vi "Image path to image refnum.vi"(7 "Image to Add [ ]":T2 {"Scale" format="%#_g %"}, 11 "error in (no error)":errorcluster) -> (8 "Image to Add refnum [ ]":T1, 15 "error out":errorcluster)   [LabVIEW 2019, in "Exaprom PDF.lvlib"]
doc: "Version 1.0\nDeveloped by Jean-Marc Simard\nCopyright © 2010, Exaprom Inc.\nAll rights reserved.\nLicense: BSD\n\nWith iTextSharp 4.1.6 (http://itextsharp.sourceforge.net)\nunder Mozilla Public License Version 1.1\n(http://www.mozilla.org/MPL/MPL-1.1.html)"
uses:
  Controls/General Controls/Image to Add [ ].ctl
  Controls/Image Controls/Image Scale.ctl
  Controls/General Controls/Image to Add refnum [ ].ctl
  C:/work/niobrara_lv/labview pdf writer fixing/DLL/itextsharp.dll
  DLL/itextsharp.dll
  Exaprom PDF.lvlib
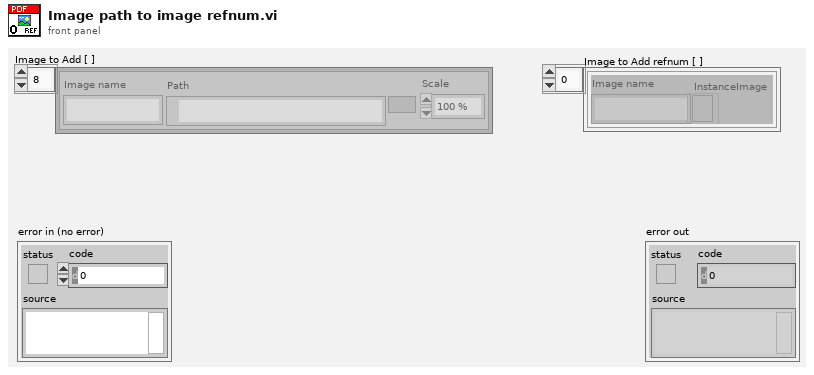
[diagram p1: front panel]
types:
  T1 = typedef "Exaprom PDF.lvlib/Image to Add refnum [ ].ctl" = cluster{"Image name":string, "InstanceImage":refnum<k24>}[]
  T2 = typedef "Exaprom PDF.lvlib/Image to Add [ ].ctl" = cluster{"Image name":string, "Path":path, "Scale":T3}[]
  T3 = typedef "Exaprom PDF.lvlib/Image Scale.ctl" = sgl
  T4 = cluster{"Image name":string, "InstanceImage":refnum<k24>}[]
  T5 = cluster{"Image name":string, "GetInstance":refnum<k24>}
  T6 = cluster{"Image name":string, "GetInstance":refnum<k24>}[]
  T7 = cluster{"Image name":string, "image":refnum<k24>}[]
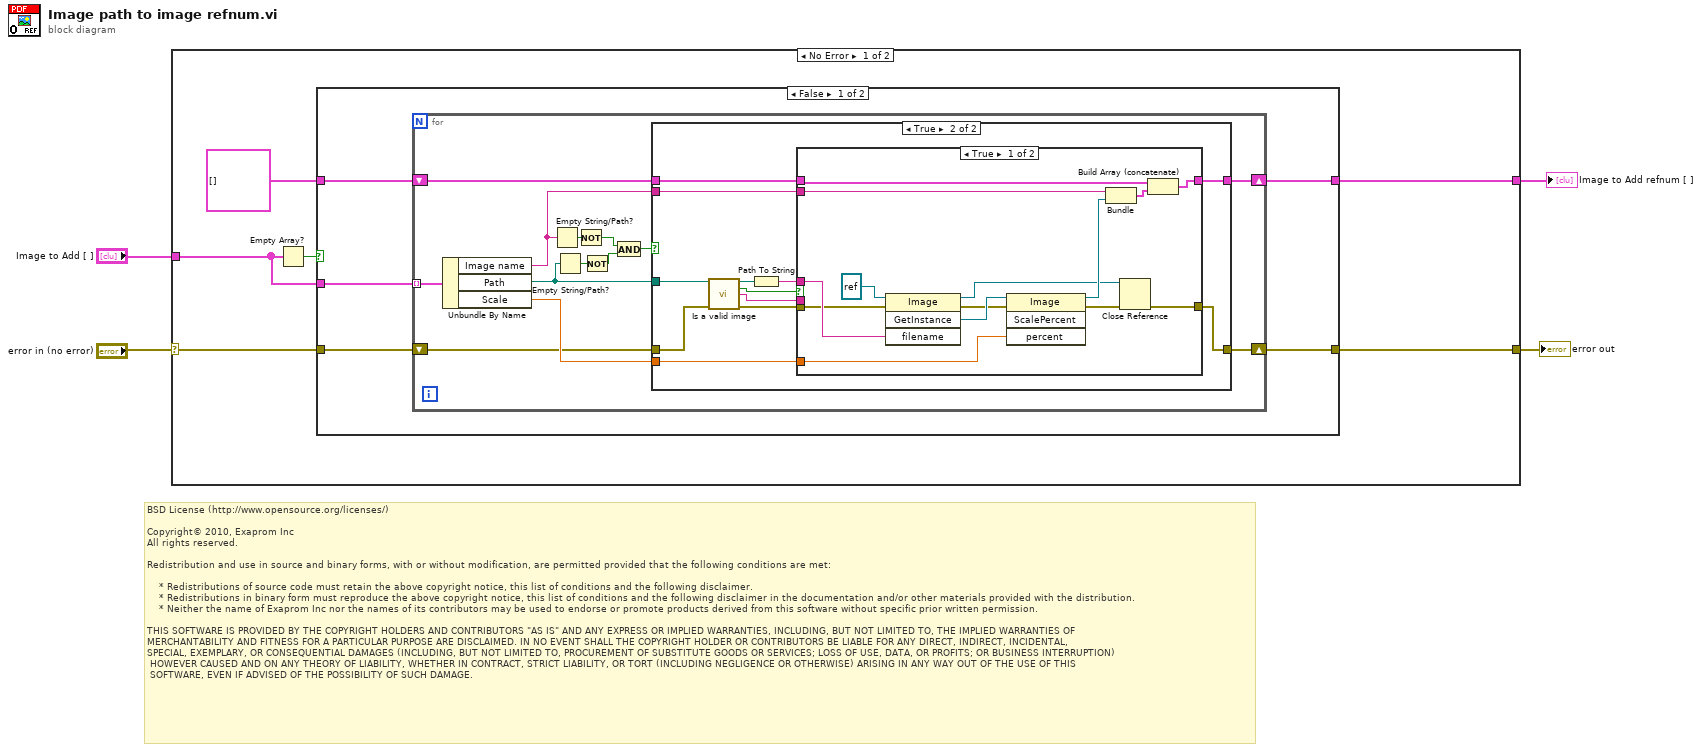
[diagram p0: block diagram]
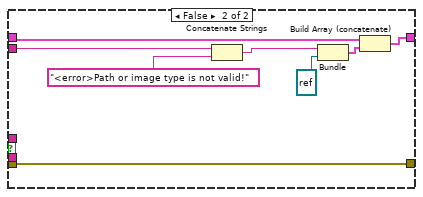
[diagram p3: hidden frame]
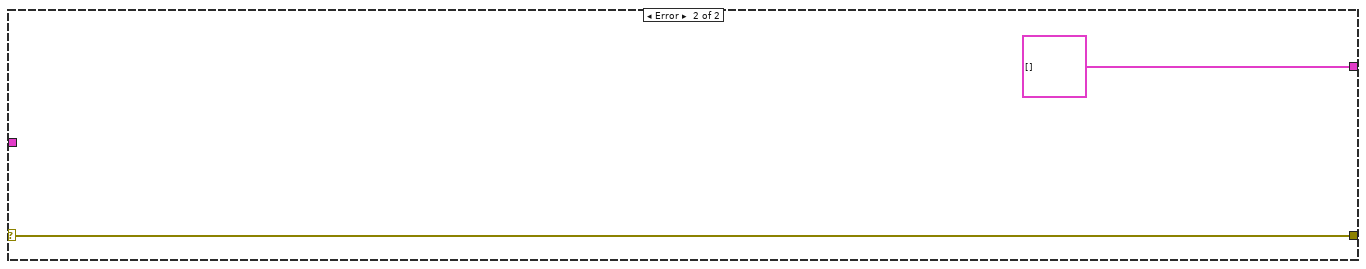
[diagram p5: hidden frame]
diagram:
  # "BSD License (http://www.opensource.org/licenses/)\n\nCopyright© 2010, Exaprom Inc\nAll rights reserved.\n\nRedistribution and use in source and binary forms, with or without modification, are permitted provided that the following conditions are met:\n\n    * Redistributions of source code must retain the above copyright notice, this list of conditions and the following disclaimer.\n    * Redistributions in binary form must reproduce the above copyright notice, this list of conditions and the following disclaimer in the documentation and/or other materials provided with the distribution.\n    * Neither the name of Exaprom Inc nor the names of its contributors may be used to endorse or promote products derived from this software without specific prior written permission.\n\nTHIS SOFTWARE IS PROVIDED BY THE COPYRIGHT HOLDERS AND CONTRIBUTORS \"AS IS\" AND ANY EXPRESS OR IMPLIED WARRANTIES, INCLUDING, BUT NOT LIMITED TO, THE IMPLIED WARRANTIES OF \nMERCHANTABILITY AND FITNESS FOR A PARTICULAR PURPOSE ARE DISCLAIMED. IN NO EVENT SHALL THE COPYRIGHT HOLDER OR CONTRIBUTORS BE LIABLE FOR ANY DIRECT, INDIRECT, INCIDENTAL,\nSPECIAL, EXEMPLARY, OR CONSEQUENTIAL DAMAGES (INCLUDING, BUT NOT LIMITED TO, PROCUREMENT OF SUBSTITUTE GOODS OR SERVICES; LOSS OF USE, DATA, OR PROFITS; OR BUSINESS INTERRUPTION)\n HOWEVER CAUSED AND ON ANY THEORY OF LIABILITY, WHETHER IN CONTRACT, STRICT LIABILITY, OR TORT (INCLUDING NEGLIGENCE OR OTHERWISE) ARISING IN ANY WAY OUT OF THE USE OF THIS\n SOFTWARE, EVEN IF ADVISED OF THE POSSIBILITY OF SUCH DAMAGE."
  n1 = case shown="No Error" "error in (no error)" {
    selector: "error in (no error)" -> [w5 w68]
    tunnel: "Image to Add [ ]" -> [w8 _]
    tunnel: [w7 w68] -> w2
    tunnel: [w6 T4 [] ("Image to Add [ ]")] -> w1
    frame No Error {
      n2 = Empty Array?(array=w8) -> (empty?=w9:bool)
      n3 = case shown="False" w9 {
        tunnel: w8 -> [w15 _]
        tunnel: T4 [] ("Image to Add [ ]") -> [w14 w66]
        tunnel: [w13 w66] -> w6
        tunnel: [w12 w65] -> w7
        tunnel: w5 -> [w11 w65]
        frame False {
          n4 = for {
            tunnel: w15 -> [w28] mode=indexing
            shift-right: [w21] -> w13
            shift-left: w14 -> [w22]
            shift-right: [w19] -> w12
            shift-left: w11 -> [w20]
            n5 = Unbundle By Name(w28) -> ("Image name"=w18:string, "Path"=w27:path, "Scale"=w23:T3)
            n6 = Empty String/Path?(string/path=w18) -> (empty?=w25:bool)
            n7 = Empty String/Path?(string/path=w27) -> (empty?=w26:bool)
            n8 = Not(x=w25) -> (.not. x?=w17:bool)
            n9 = Not(x=w26) -> (.not. x?=w16:bool)
            n10 = And(x=w17, y=w16) -> (x .and. y?=w24:bool)
            n11 = case shown="True" w24 {
              tunnel: w27 -> [_ w41]
              tunnel: w23 -> [_ w39]
              tunnel: w22 -> [w30 w37]
              tunnel: [w30 w36] -> w21
              tunnel: w20 -> [w29 w31]
              tunnel: [w29 w38] -> w19
              tunnel: w18 -> [_ w35]
              frame False {
              }
              frame True {
                n12 = call "Is a valid image.vi"("Image path"=w41, "error in (no error)"=w31) -> ("dup path"=w42:path, "Valid Image?"=w33:bool, "Message"=w32:string, "error out"=w34:errorcluster)  [unwired: 10 out]
                n13 = Path To String(path=w42) -> (string=w40:string)
                n14 = case shown="True" w33 {
                  tunnel: w40 -> [w54 _]
                  tunnel: w39 -> [w53 _]
                  tunnel: [w46 w60] -> w38
                  tunnel: w37 -> [w52 w64]
                  tunnel: [w51 w63] -> w36
                  tunnel: w35 -> [w49 w62]
                  tunnel: w34 -> [w43 w60]
                  tunnel: w32 -> [_ _]
                  frame True {
                    n15 = invoke class="Image" method="GetInstance"(reference=refnum<k24> refnum ("image"), error in=w43, "filename"=w54) -> (reference out=w45:refnum<k24>, error out=w55:errorcluster, "GetInstance"=w56:refnum<k24>)  [unwired: 1 in, 1 out]
                    n16 = invoke class="Image" method="ScalePercent"(reference=w56, error in=w55, "percent"=w53) -> (reference out=w50:refnum<k24>, error out=w47:errorcluster)  [unwired: 1 in, 2 out]
                    n17 = Bundle("Image name"=w49, "GetInstance"=w50) -> (w48:T5)  [unwired: 1 out]
                    n18 = Close Reference(reference=w45, error in (no error)=w47) -> (error out=w46:errorcluster)
                    n19 = Build Array (concatenate)(w52, w48) -> (w51:T6)
                  }
                  frame False {
                    n20 = Concatenate Strings(w62, "<error>Path or image type is not valid!") -> (w59:string)
                    n21 = Bundle(w59, "image"=refnum<k24> refnum) -> (w61:cluster{string, "image":refnum<k24>})  [unwired: 1 out]
                    n22 = Build Array (concatenate)(w64, w61) -> (w63:T7)
                  }
                }
              }
            }
          }
        }
        frame True {
        }
      }
    }
    frame Error {
    }
  }
  "error out" <- w2
  "Image to Add refnum [ ]" <- w1
